vi "全局 1.vi"() -> ()   [LabVIEW 2018]
panel:
  in  "数值":dbl
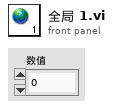
[diagram p1: front panel]
diagram:
